vi "Wake HL.vi"(8 "error in (no error)":errorcluster, 10 "event data":T2, 11 "User events":T1) -> (0 "error out":errorcluster)   [LabVIEW 2020, in "NI DAQ.lvlib"]
uses:
  NI DAQ.lvlib
  Continuous aquisition params.ctl
  Task list.ctl
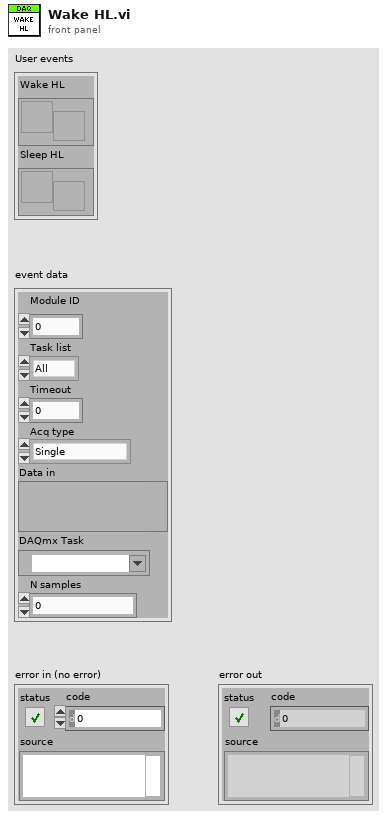
[diagram p1: front panel]
types:
  T1 = cluster{"Wake HL":refnum<user-event>, "Sleep HL":refnum<user-event>}
  T2 = typedef "NI DAQ.lvlib/Continuous aquisition params.ctl" = cluster{"Module ID":i32, "Task list":T3, "Timeout":i32, "Acq type":enum16{"Single", "Multiple"}, "Data in":variant, "DAQmx Task":refnum<k21>, "N samples":i32}
  T3 = typedef "NI DAQ.lvlib/Task list.ctl" = enum16{"All", "DO task", "DI task", "AO task", "AI task"}
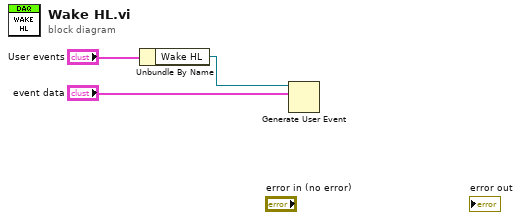
[diagram p0: block diagram]
diagram:
  n1 = Unbundle By Name("User events") -> ("Wake HL"=w2:refnum<user-event>)
  n2 = Generate User Event(user event=w2, event data cluster="event data") -> ()  [unwired: 2 in, 2 out]
